vi "Rotate.vi"(0 "Angle (Rad)":dbl, 1 "Execute":bool, 2 "Speed (0-1)":dbl) -> (4 "Done Executing":bool)   [LabVIEW 2011]
uses:
  Controls/Robot Orientation.ctl
  <vilib>/Rock Robotics/WPI/CAN/Jaguar/SubVIs/WPI_CANJaguar_StatusSelect.ctl
  Globals/Robot Radii.vi
  Globals/Robot Jaguars.vi
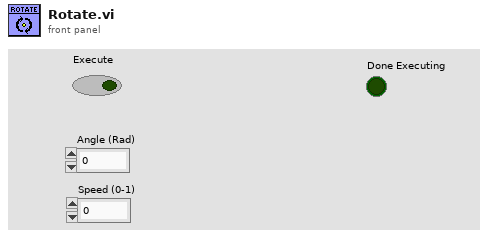
[diagram p1: front panel]
types:
  T1 = typedef "Robot Orientation.ctl" = enum16{"Landscape", "Portrait"}
  T2 = typedef "WPI_CANJaguar_StatusSelect.ctl" = enum16{"Output Percent VBus", "Output Voltage", "Bus Voltage", "Current", "Temperature", "Position", "Speed", "Limit Switches", "Faults", "Fault Counters", "Power Cycle"}
  T3 = typedef "WPI_MotorControlDeviceRef.ctl" = cluster{"DeviceStatus":errorcluster, "Type":enum16{"PWM", "CAN"}, "PWM":cluster{"Digital Module":T4, "PWM Channel":T5, "DeadBand":T6}, "CAN":cluster{"Device Number":u8, "Control Mode":T7, "Semaphore":T8, "Max Vout":dbl}, "Invert":bool, "TransformRef":T9, "InvTransformRef":T9}
  T4 = typedef "FPGA_TypedefDigitalModule.ctl" = enum16{"Digital Module 1", "Digital Module 2"}
  T5 = typedef "FPGA_DIOPWMChannel.ctl" = enum8{"PWM 1", "PWM 2", "PWM 3", "PWM 4", "PWM 5", "PWM 6", "PWM 7", "PWM 8", "PWM 9", "PWM 10", "Invalid"}
  T6 = typedef "WPI_PWMDeadband.ctl" = cluster{"Name":string, "maxPositivePwm":i32, "minPositivePwm":i32, "centerPwm":i32, "maxNegativePwm":i32, "minNegativePwm":i32, "angularRange":u16}
  T7 = typedef "WPI_CANJaguar_ControlMode.ctl" = enum8{"Percent VBus", "Current", "Speed", "Position", "Voltage"}
  T8 = typedef "Semaphore RefNum" = refnum<k1>
  T9 = typedef "WPI_PWMTransform_ConPane.ctl" = refnum<vi>
  T10 = cluster{"Front Left Drive":T3, "Front Right Drive":T3, "Rear Left Drive":T3, "Rear Right Drive":T3, "Front Left Steer":T3, "Front Right Steer":T3, "Rear Left Steer":T3, "Rear Right Steer":T3}
  T11 = typedef "WPI_CANJaguar_Status.ctl" = cluster{"Output Percent VBus":dbl, "Output Voltage":dbl, "Bus Voltage":dbl, "Current":dbl, "Temperature":dbl, "Position":dbl, "Speed":dbl, "Limits":cluster{"Forward Limit":bool, "Reverse Limit":bool, "Forward Soft Limit":bool, "Reverse Soft Limit":bool, "Sticky Forward Limit":bool, "Sticky Reverse Limit":bool, "Sticky Forward Soft Limit":bool, "Sticky Reverse Soft Limit":bool}, "Faults":cluster{"Current Fault":bool, "Temperature Fault":bool, "Bus Voltage Fault":bool, "Gate Driver Fault":bool, "Comm Fault":bool}, "Fault Counters":cluster{"Current Faults":u8, "Temperature Faults":u8, "Bus Voltage Faults":u8, "Gate Driver Faults":u8, "Comm Faults":u8, "CAN Status":u8, "CAN RX Errors":u8, "CAN TX Errors":u8}, "Power Cycle":bool}
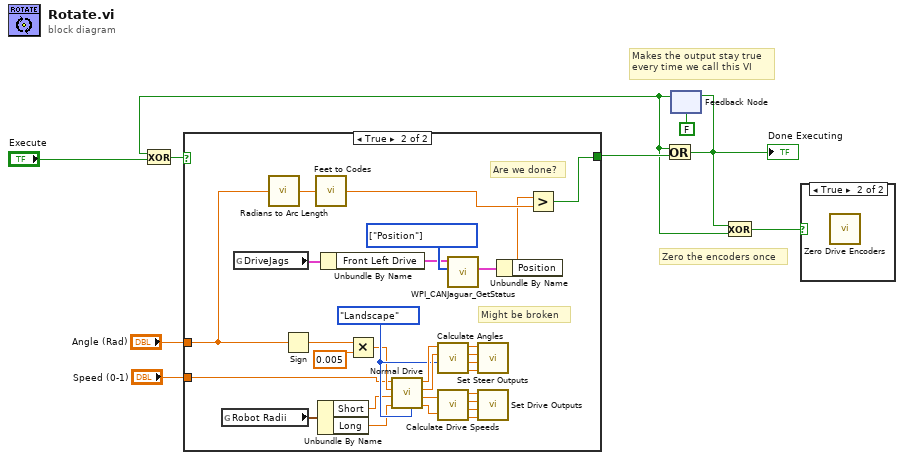
[diagram p0: block diagram]
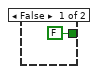
[diagram p3: hidden frame]
diagram:
  # "Makes the output stay true\nevery time we call this VI"
  # "Zero the encoders once"
  n1 = feedback #1(FALSE) -> (w2:bool)
  n2 = Exclusive Or(1:"Execute", 2:w2) -> (0:w9:bool)
  n3 = case shown="True" w9 {
    tunnel: [FALSE w39] -> w7
    tunnel: "Angle (Rad)" -> [_ w11]
    tunnel: "Speed (0-1)" -> [_ w13]
    frame False {
    }
    frame True {
      w20 = Robot_Orientation."Landscape" ("Robot Orientation")
      w37 = T2[] [enum."Position"] items=["Output Percent VBus", "Output Voltage", "Bus Voltage", "Current", "Temperature", "Position", "Speed", "Limit Switches", "Faults", "Fault Counters", "Power Cycle"] ("Status Select")
      # "Might be broken"
      # "Are we done?"
      n4 = global read "Robot Radii.vi" "Robot Radii"() -> (w19:cluster{"Short":dbl, "Long":dbl})
      n5 = global read "Robot Jaguars.vi" "DriveJags"() -> (w34:T10)
      n6 = call "Radians to Arc Length.vi"("Angle (Radians)"=w11) -> ("Arc Length (Feet)"=w12:dbl)
      n7 = Sign(1:w11) -> (0:w16:dbl)
      n8 = call "Feet to Codes.vi"("Feet"=w12) -> ("Codes"=w38:dbl)
      n9 = Unbundle By Name(w19) -> ("Short"=w18:dbl, "Long"=w17:dbl)
      n10 = Unbundle By Name(w34) -> ("Front Left Drive"=w33:T3)
      n11 = Multiply(x=w16, y=0.005) -> (x*y=w14:dbl)
      n12 = call "Normal Drive.vi"("Joy X"=w13, "Joy Y"=w14, "Short Radius (Inches)"=w18, "Long Radius (Inches)"=w17, "Robot Orientation"=w20) -> ("Front Left Angle Out"=w22:dbl, "Front Right Angle Out"=w21:dbl, "Left Speed Out"=w24:dbl, "Right Speed Out"=w23:dbl)  [unwired: 1 in]
      n13 = call "Calculate Angles.vi"("Robot Orientation"=w20, "Right Angle In"=w21, "Left Angle In"=w22) -> ("Rear Right Steer Out"=w25:dbl, "Rear Left Pot Out"=w26:dbl, "Front Right Pot Out"=w27:dbl, "Front Left Pot Out"=w28:dbl)  [unwired: 1 in]
      n14 = call "Calculate Drive Speeds.vi"("Left Speed In"=w24, "Right Speed In"=w23) -> ("Front Left Speed"=w32:dbl, "Front Right Speed"=w30:dbl, "Rear Left Speed"=w31:dbl, "Rear Right Speed"=w29:dbl)  [unwired: 2 in]
      n15 = call <vilib>:"WPI_CANJaguar_GetStatus.vi"("Status Select"=w37, "CAN Jaguar Ref"=w33) -> ("Status"=w36:T11)  [unwired: 7 in, 2 out]
      n16 = call "Set Steer Outputs.vi"("Rear Right"=w25, "Rear Left"=w26, "Front Right"=w27, "Front Left"=w28) -> ()  [unwired: 8 in]
      n17 = call "Set Drive Outputs.vi"("Rear Right"=w29, "Rear Left"=w30, "Front Right"=w31, "Front Left"=w32) -> ()  [unwired: 8 in]
      n18 = Unbundle By Name(w36) -> ("Position"=w35:dbl)
      n19 = Greater?(x=w35, y=w38) -> (0:w39:bool)
    }
  }
  n20 = Or(x=w2, y=w7) -> (x .or. y?=w1:bool)
  "Done Executing" <- w1
  n21 = feedback-in #1(w1) -> ()
  n22 = Exclusive Or(1:w2, 2:w1) -> (0:w3:bool)
  n23 = case shown="True" w3 {
    frame False {
    }
    frame True {
      n24 = call "Zero Drive Encoders.vi"() -> ()  [unwired: 12 in]
    }
  }
